vi "EvaluateBoolExpression.vi"(8 "error in (no error)":errorcluster, 11 "infix expression":string) -> (0 "error out":errorcluster, 3 "result":bool)   [LabVIEW 2017, in "ExpressionEvaluator.lvlib"]
uses:
  <vilib>/addons/InsightCM/Utilities/ExpressionEvaluator/ExpressionEvaluator.lvlib
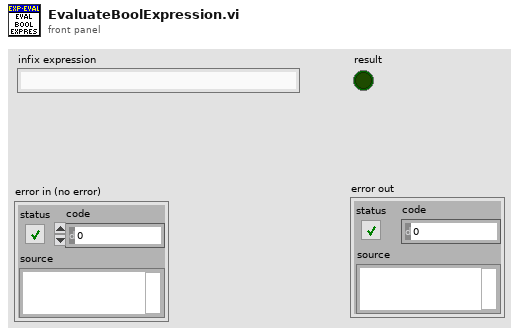
[diagram p1: front panel]
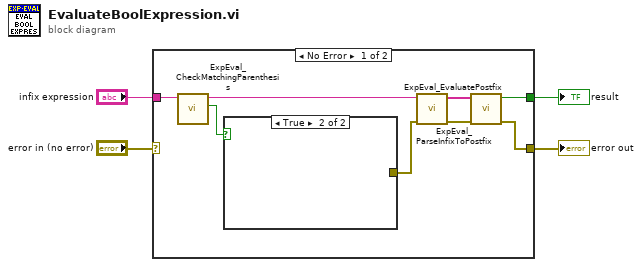
[diagram p0: block diagram]
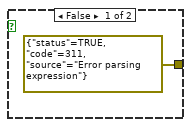
[diagram p2: hidden frame]
diagram:
  n1 = case shown="No Error" "error in (no error)" {
    selector: "error in (no error)" -> [_ w14]
    tunnel: [w10 w14] -> w4
    tunnel: [w9 _] -> w3
    tunnel: "infix expression" -> [w7 _]
    frame No Error {
      n2 = call <vilib>:"ExpEval_CheckMatchingParenthesis.vi"("expression in"=w7) -> ("match"=w5:bool, "expression out"=w6:string)  [unwired: 9 in]
      n3 = case shown="True" w5 {
        tunnel: [errorcluster {"status"=TRUE, "code"=311, "source"="Error parsing expression"} ("error constant") _] -> w8
        frame False {
        }
        frame True {
        }
      }
      n4 = call <vilib>:"ExpEval_ParseInfixToPostfix.vi"("error in (no error)"=w8, "infix expression"=w6) -> ("error out"=w11:errorcluster, "postfix array"=w12:string[])  [unwired: 8 in]
      n5 = call <vilib>:"ExpEval_EvaluatePostfix.vi"("error in (no error)"=w11, "postfix array"=w12) -> ("error out"=w10:errorcluster, "result"=w9:bool)  [unwired: 8 in]
    }
    frame Error {
    }
  }
  "error out" <- w4
  "result" <- w3
